vi "CS_Initialize.vi"() -> ()   [LabVIEW 2013, in "LightField Automation.lvclass"]
uses:
  LightField Automation.lvclass
  CS_LFAClassGlobal.vi
panel:
  in  "stop":bool
  in  "Is Visible?":bool=TRUE
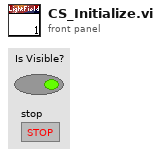
[diagram p1: front panel]
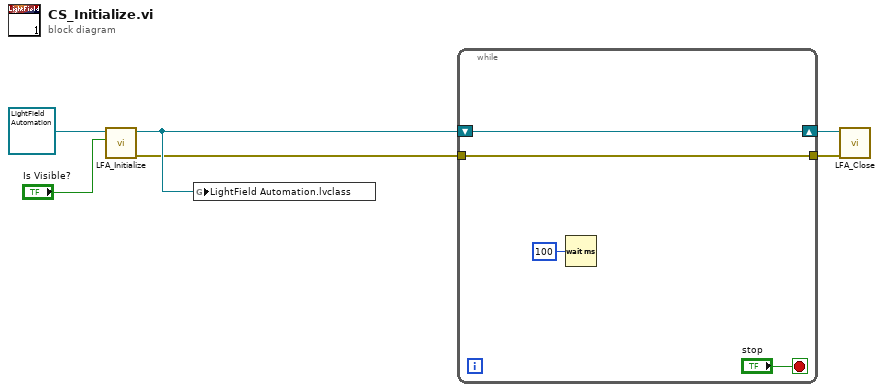
[diagram p0: block diagram]
diagram:
  n1 = call "LFA_Initialize.vi"("Is Visible?"="Is Visible?", "LightField Automation in"=refnum<class "LightField Automation.lvclass"> refnum ("LightField Automation.lvclass")) -> ("error out"=w2:errorcluster, "LightField Automation out"=w4:refnum<class "LightField Automation.lvclass">)  [unwired: 8 in]
  n2 = global write "CS_LFAClassGlobal.vi" "LightField Automation.lvclass"(w4) -> ()
  n3 = while {
    shift-right: [w9] -> w3
    shift-left: w4 -> [w9]
    tunnel: w2 -> [w8]
    tunnel: [w8] -> w1
    stop <- "stop" stop-if-true
    n4 = Wait (ms)(milliseconds to wait=u32 100) -> ()  [unwired: 1 out]
  }
  n5 = call "LFA_Close.vi"("error in (no error)"=w1, "LightField Automation in"=w3) -> ()  [unwired: 8 in, 2 out]
